vi "Init 1.vi"(3 "Container State":T4, 4 "Previous State":variant, 5 "Previous Version":T3) -> (2 "Current State":T1)   [LabVIEW 2012, in "paint Xcontrol.xctl"]
doc: "This VI initializes the display state of the Paint XControl when you first place the XControl or when a VI containing the control is loaded into memory.\n\nUse this VI to handle versioning of XControls. You can update XControl instances saved in a previous version by converting the state from an older format to the current one.\n\nAllocate any resources needed by the XControl here. The resources can then be deallocated in the UnInit ability."
uses:
  paint Xcontrol.xctl
  State 1.ctl
  controls/tool enum.ctl
  <vilib>/_xctls/Container State.ctl
  <vilib>/_xctls/Version.ctl
  <vilib>/_xctls/XControlSupport.lvlib
panel:
  in  "Default Indicator State":T1
  in  "Default Control State":T1
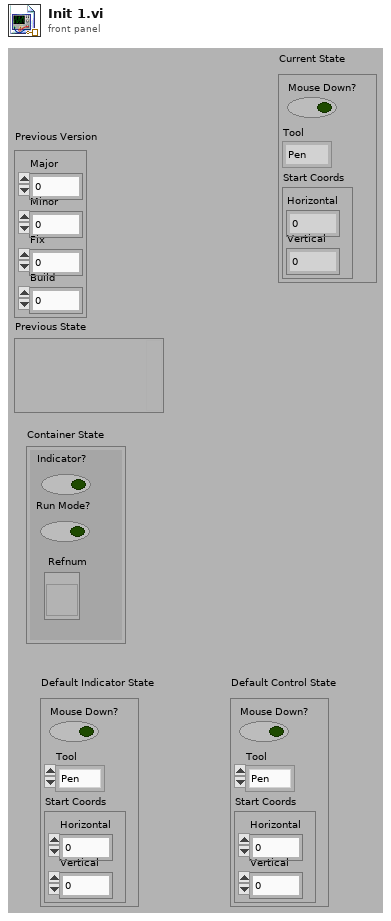
[diagram p1: front panel]
types:
  T1 = typedef "paint Xcontrol.xctl/State 1.ctl" = cluster{"Mouse Down?":bool, "Tool":T2, "Start Coords":cluster{"Horizontal":i32, "Vertical":i32}}
  T2 = typedef "paint Xcontrol.xctl/tool enum.ctl" = enum16{"Pen", "Square", "Circle", "Text", "Line"}
  T3 = typedef "XControlSupport.lvlib/Version.ctl" = cluster{"Major":u16, "Minor":u16, "Fix":u16, "Build":u16}
  T4 = typedef "XControlSupport.lvlib/Container State.ctl" = cluster{"Indicator?":bool, "Run Mode?":bool, " Refnum":refnum<vi>}
  T5 = cluster{"Major":u16, "Minor":u16, "Fix":u16, "Build":u16}
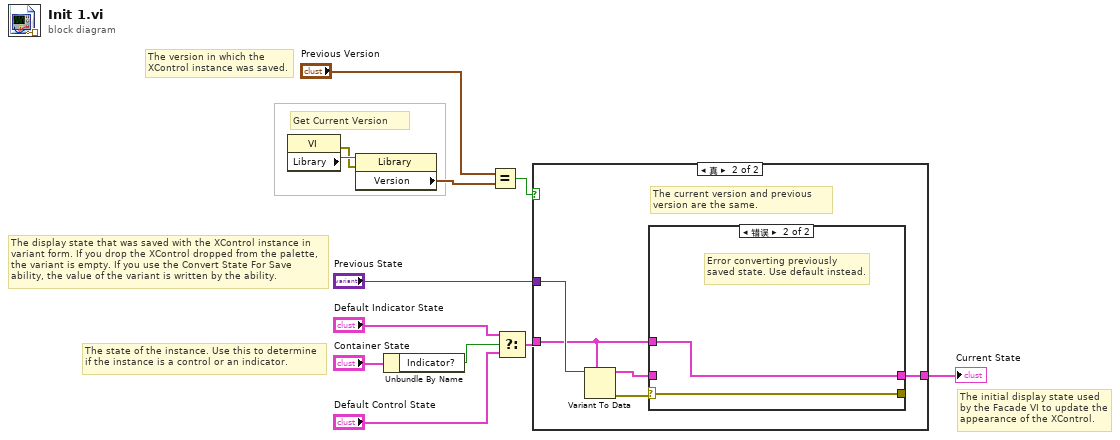
[diagram p0: block diagram]
diagram:
  # "The initial display state used by the Facade VI to update the appearance of the XControl."
  # "The state of the instance. Use this to determine if the instance is a control or an indicator."
  # "The display state that was saved with the XControl instance in variant form. If you drop the XControl dropped from the palette, the variant is empty. If you use the Convert State For Save ability, the value of the variant is written by the ability."
  # "The version in which the XControl instance was saved."
  # "Get Current Version"
  n1 = property class="VI"() -> (error out=w2:errorcluster, "Library"=w3:refnum<vi>)  [unwired: 2 in, 1 out]
  n2 = property class="Library"(reference=w3, error in=w2) -> ("Version"=w1:T5)  [unwired: 2 out]
  n3 = Unbundle By Name("Container State") -> ("Indicator?"=w5:bool)
  n4 = Equal?(x="Previous Version", y=w1) -> (x = y?=w11:bool)
  n5 = Select(t="Default Indicator State", s=w5, f="Default Control State") -> (s? t:f=w4:T1)
  n6 = case shown="真" w11 {
    tunnel: "Previous State" -> [_ w18]
    tunnel: [w13 w14] -> w9
    tunnel: w4 -> [w13 w15]
    frame False {
      # "Convert from a previous version."
    }
    frame True {
      # "The current version and previous version are the same."
      n7 = Variant To Data(type=w15, Variant=w18) -> (data=w16:T1, error out=w17:errorcluster)  [unwired: 1 in]
      n8 = case shown="错误" w17 {
        selector: w17 -> [w20 w21]
        tunnel: w16 -> [w19 _]
        tunnel: [w19 w22] -> w14
        tunnel: w15 -> [_ w22]
        tunnel: [w20 w21] -> _
        frame No Error {
        }
        frame Error {
          # "Error converting previously \nsaved state. Use default instead."
        }
      }
    }
  }
  "Current State" <- w9
